vi "FPGA Main.vi"() -> ()   [LabVIEW 2022 SP3]
uses:
  <vilib>/rvi/Emulation/niFpgaGetClockAttributes.vi
  <vilib>/rvi/Emulation/niFpgaSctlEmulationGetInTimedLoop.vi
  <vilib>/rvi/Emulation/niFpgaEmulationReportErrorSimple.vi
  <vilib>/rvi/eio/common/nirviEmuTemplateMethod_errors.vi
  <vilib>/rvi/Emulation/niFpgaCriticalErrorInLSC.vi
  <vilib>/eio/EIONode/EIONode.xnode
panel:
  out "USER Push Button":bool
  in  "USER FPGA LED":u8
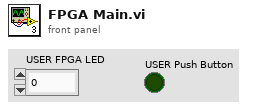
[diagram p1: front panel]
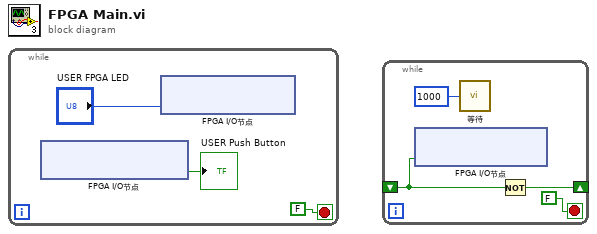
[diagram p0: block diagram]
diagram:
  n1 = while {
    stop <- FALSE stop-if-true
    n2 = xnode "FPGA I/O节点"() -> ("USER Push Button"=→"USER Push Button":bool)  [unwired: 1 in, 1 out]
    n3 = xnode "FPGA I/O节点"("USER FPGA LED"="USER FPGA LED") -> ()  [unwired: 1 in, 1 out]
  }
  n4 = while {
    shift-right: [w7] -> _
    shift-left: _ -> [w6]
    stop <- FALSE stop-if-true
    n5 = xnode "FPGA I/O节点"("模块7/User LED"=w6) -> ()  [unwired: 1 in, 1 out]
    n6 = call "等待"("Count(mSec)"=u32 1000) -> ()  [unwired: 1 out]
    n7 = Not(x=w6) -> (.not. x?=w7:bool)
  }
